vi "LogTimeStamp.vi"(8 "error in (no error)":errorcluster, 10 "New Image":T1, 11 "GRMActor in":refnum<class "DataLoggerUI.lvclass">) -> (0 "error out":errorcluster, 2 "Image Out":T1, 3 "GRMActor out":refnum<class "DataLoggerUI.lvclass">)   [LabVIEW 2020, in "DataLogger.lvlib" / "DataLoggerUI.lvlib" / "DataLoggerUI.lvclass"]
uses:
  DataLoggerUI/DataLoggerUI.lvclass
  <vilib>/vision/Image Controls.llb/IMAQ Image.ctl
  DataLoggerUI/DataLoggerUI.lvclass/DataLoggerUI.ctl
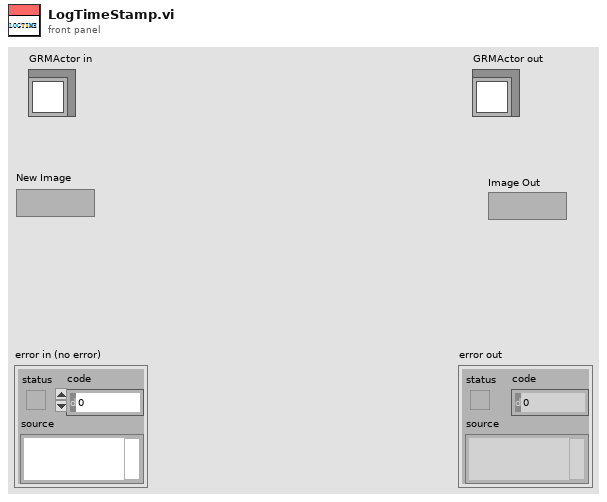
[diagram p1: front panel]
types:
  T1 = typedef "IMAQ Image.ctl" = refnum<image>
  T2 = cluster{"Values[0]":string, "Values[1]":string, "Values[2]":string, "Values[3]":string, "Values[4]":string, "Values[5]":string, "Values[6]":string, "Values[7]":string, "Values[8]":string, "Values[9]":string, "Values[10]":string, "Values[11]":string, "Values[12]":string}
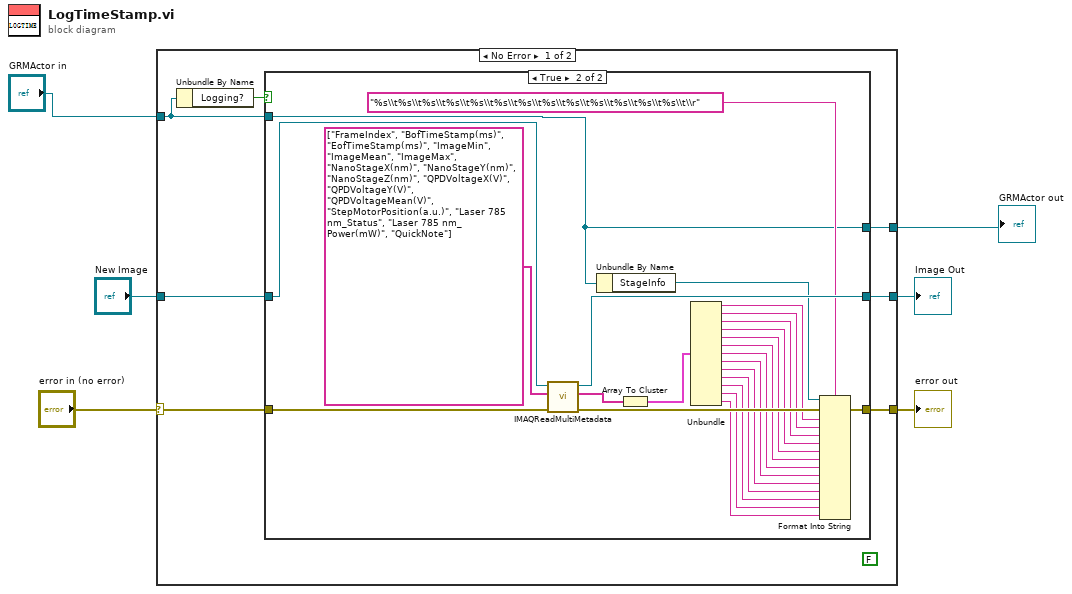
[diagram p0: block diagram]
diagram:
  n1 = case shown="No Error" "error in (no error)" {
    selector: "error in (no error)" -> [w13 w43]
    tunnel: [w10 w43] -> w5
    tunnel: [w9 w42] -> w1
    tunnel: "GRMActor in" -> [w8 w42]
    tunnel: "New Image" -> [w12 w41]
    tunnel: [w11 w41] -> w3
    frame No Error {
      (unwired) FALSE ("LogQuickNote")
      n2 = Unbundle By Name(w8) -> ("Logging?"=w7:bool)
      n3 = case shown="True" w7 {
        tunnel: w13 -> [w14 w40]
        tunnel: w8 -> [w15 w17]
        tunnel: w12 -> [w16 w39]
        tunnel: [w16 w38] -> w11
        tunnel: [w14 w36] -> w10
        tunnel: [w15 w17] -> w9
        frame False {
        }
        frame True {
          n4 = call "IMAQReadMultiMetadata.vi"("error in (no error)"=w40, "Keys"=string[] ["FrameIndex", "BofTimeStamp(ms)", "EofTimeStamp(ms)", "ImageMin", "ImageMean", "ImageMax", "NanoStageX(nm)", "NanoStageY(nm)", "NanoStageZ(nm)", "QPDVoltageX(V)", "QPDVoltageY(V)", "QPDVoltageMean(V)", "StepMotorPosition(a.u.)", "Laser 785 nm_Status", "Laser 785 nm_Power(mW)", "QuickNote"], "Image In"=w39) -> ("error out"=w37:errorcluster, "Values"=w33:string[], "Image Out"=w38:T1)  [unwired: 6 in]
          n5 = Unbundle By Name(w17) -> ("StageInfo"=w35:refnum<file>)
          n6 = Array To Cluster(array=w33) -> (cluster=w32:T2)
          n7 = Unbundle(w32) -> ("Values[0]"=w31:string, "Values[1]"=w30:string, "Values[2]"=w29:string, "Values[3]"=w28:string, "Values[4]"=w27:string, "Values[5]"=w26:string, "Values[6]"=w25:string, "Values[7]"=w24:string, "Values[8]"=w23:string, "Values[9]"=w22:string, "Values[10]"=w21:string, "Values[11]"=w20:string, "Values[12]"=w18:string)
          n8 = Format Into String(format string="%s\\t%s\\t%s\\t%s\\t%s\\t%s\\t%s\\t%s\\t%s\\t%s\\t%s\\t%s\\t%s\\t\\r", initial string=w35, error in=w37, w31, w30, w29, w28, w27, w26, w25, w24, w23, w22, w21, w20, w18) -> (error out=w36:errorcluster)  [unwired: 1 out]
        }
      }
    }
    frame Error {
    }
  }
  "error out" <- w5
  "Image Out" <- w3
  "GRMActor out" <- w1
